vi "dat_fuses.vi"(2 "fuse_av_2-Ready for Output":bool, 3 "fuse_av_1-Ready for Output":bool) -> (0 "fuse_av_2":T1, 1 "fuse_av_1":T1)   [LabVIEW 2018]
uses:
  validated_bool.ctl
  <vilib>/rvi/DataTransferAndStorage/Container/Common/niFpgaContainerExecOnDevCompGetState.vi
  <vilib>/rvi/Emulation/niFpgaEmulationIsFPGAContextNoSignature.vi
  <vilib>/rvi/Emulation/niFpgaSctlEmulationGetInTimedLoop.vi
  <vilib>/rvi/errors/niFpgaSetErrorForExecOnDevCompSimple.vi
  <vilib>/rvi/eio/common/nirviEmuReportErrorAndStop.vi
  <vilib>/rvi/DataTransferAndStorage/Container/Common/niFpgaContainerGetUniqueNameForEmu.vi
  <vilib>/rvi/FIFO/Fifo_Resource/nirvififoEmulationSetSize.vi
  <vilib>/rvi/FIFO/Fifo_Resource/nirviFifoEmulationQueueMgr.vi
  <instcachedir>/0/nirviFifoEmulationQueueMgr_E5CAEC123FF24DC58D834DCA3CDAA9B5.lvgen/nirviFifoEmulationQueueMgr_E5CAEC123FF24DC58D834DCA3CDAA9B5_001.vi
  <vilib>/rvi/FIFO/Fifo_Resource/nirvififoEmulationDetermineInputValidOut.vi
  <vilib>/rvi/FIFO/Fifo_Resource/nirvififoEmulationCreateLock.vi
  <vilib>/rvi/Emulation/niFpgaProcessEmulError.vi
  <vilib>/rvi/FIFO/Fifo_Resource/nirvififoEmulationObtainLock.vi
  <vilib>/rvi/FIFO/Fifo_Resource/nirvififoEmulationReleaseLock.vi
  <vilib>/rvi/occurrence/nirviWaitOnOccurrenceBase.vi
  <vilib>/rvi/errors/nirviReportUnexpectedCaseInternalError.vi
  <vilib>/rvi/errors/nirviReportUnexpectedCaseInternalError (U32).vi
  <vilib>/Utility/error.llb/Clear Errors.vi
  <vilib>/rvi/interface/RandomDataEmulation/niFpgaRandomDataHandleErrors.vi
  <vilib>/rvi/DataTransferAndStorage/Container/XNode/niFpgaContainer.xnode
  <vilib>/rvi/FIFO/Fifo_Resource/niFpgaFifoEmulationRefIn.vi
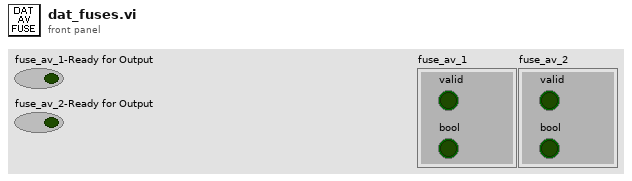
[diagram p1: front panel]
types:
  T1 = typedef "validated_bool.ctl" = cluster{"valid":bool, "bool":bool}
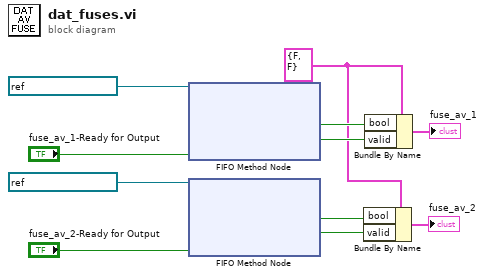
[diagram p0: block diagram]
diagram:
  w7 = T1 {"valid"=FALSE, "bool"=FALSE} ("Cluster")
  n1 = xnode ("FIFO Method Node")("Ready for Output"="fuse_av_1-Ready for Output", "FIFO In"=refnum<k21> "fuse_avionics_1") -> ("Element"=w9:bool, "Output Valid"=w8:bool)  [unwired: 1 out]
  n2 = xnode ("FIFO Method Node")("Ready for Output"="fuse_av_2-Ready for Output", "FIFO In"=refnum<k21> "fuse_avionics_2") -> ("Element"=w6:bool, "Output Valid"=w5:bool)  [unwired: 1 out]
  n3 = Bundle By Name(cluster=w7, "bool"=w6, "valid"=w5) -> (→"fuse_av_2":T1)
  n4 = Bundle By Name(cluster=w7, "bool"=w9, "valid"=w8) -> (→"fuse_av_1":T1)
